vi "ExitInstrument.vi"(8 "error in (no error)":errorcluster) -> (0 "error out":errorcluster, 3 "function return":i16)   [LabVIEW 2013, in "HS3OverallRoutines.lvlib"]
doc: "Description: Close the instrument. Free any allocated resources and memory, place the relays in their passive state, etc. Only call this routine when the instrument is no longer required\n\nInput: -\nOutput: Return value E_NO_ERRORS | E_NOT_INITIALIZED\n\nFunction prototype: word ExitInstrument( void )\n\nshort int ExitInstrument ( void );"
uses:
  HS3OverallRoutines.lvlib
  hs3.dll
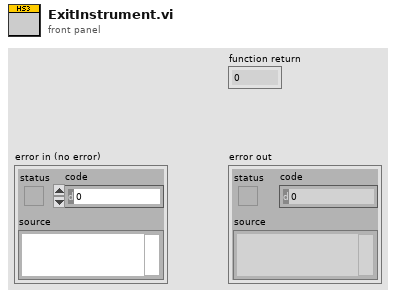
[diagram p1: front panel]
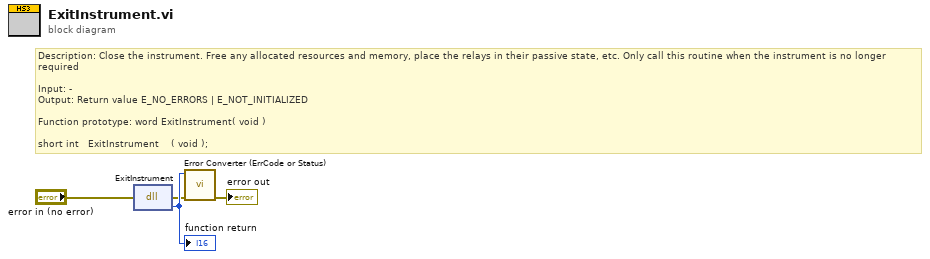
[diagram p0: block diagram]
diagram:
  # "Description: Close the instrument. Free any allocated resources and memory, place the relays in their passive state, etc. Only call this routine when the instrument is no longer required\n\nInput: -\nOutput: Return value E_NO_ERRORS | E_NOT_INITIALIZED\n\nFunction prototype: word ExitInstrument( void )\n\nshort int \t\tExitInstrument\t\t\t\t( void );"
  n1 = dll-call lib="C:/Documents and Settings/admin/Pulpit/HS3 LabViewLib/HS3_WRAPPER/OverallRoutines/hs3.*" fn="ExitInstrument"(error in="error in (no error)") -> (error out=w2:errorcluster, w4:i16)  [unwired: 2 in, 1 out]
  "function return" <- w4
  n2 = call "Error Converter (ErrCode or Status).vi"("error in (no error)"=w2, "error code"=w4) -> ("error out"=→"error out":errorcluster)  [unwired: 9 in]
